vi "Message Handler.vi"(8 "error in (no error)":errorcluster, 11 "PID Loop in":refnum<class "PID Loop.lvclass">) -> (0 "error out":errorcluster, 3 "Zero Timeout Message Handler out":refnum<class "Zero Timeout Message Handler.lvclass">)   [LabVIEW 2024, in "PID Loop.lvlib" / "PID Loop.lvclass"]
uses:
  PID Loop.lvclass
  src/Zero Timeout Message Handler/Zero Timeout Message Handler/Zero Timeout Message Handler.lvclass
  PID Loop.lvclass/PID Loop.ctl
panel:
  out "Waveform Chart":dbl(graph)
  out "dt (s)":dbl
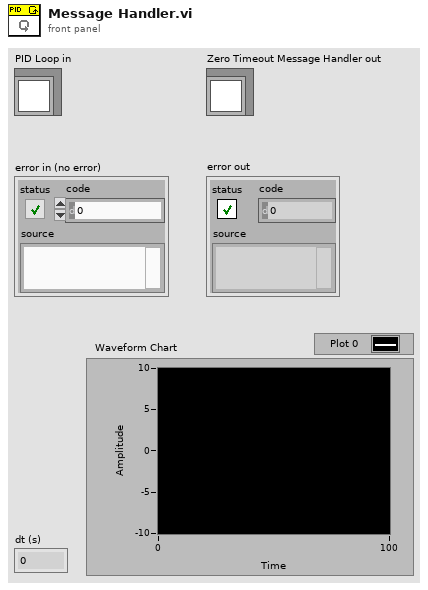
[diagram p1: front panel]
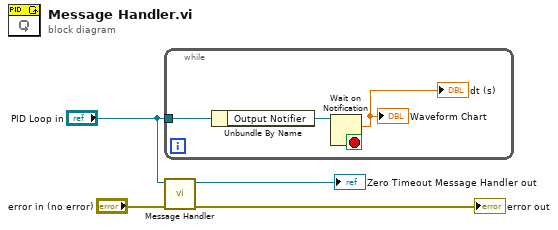
[diagram p0: block diagram]
diagram:
  n1 = while {
    tunnel: "PID Loop in" -> [w8]
    stop <- w6 stop-if-true
    n2 = Unbundle By Name(w8) -> ("Output Notifier"=w7:refnum<notifier>)
    n3 = Wait on Notification(notifier=w7) -> (notification=→"dt (s)" →"Waveform Chart":dbl, error out=w6:errorcluster)  [unwired: 3 in, 2 out]
  }
  n4 = call-parent "Message Handler.vi"("error in (no error)"="error in (no error)", "Zero Timeout Message Handler in"="PID Loop in") -> ("error out"=→"error out":errorcluster, "Zero Timeout Message Handler out"=→"Zero Timeout Message Handler out":refnum<class "Zero Timeout Message Handler.lvclass">)  [unwired: 8 in]
